vi "Paint Bounding Box.vi"(9 "Camera Image":T3) -> (0 "error out":errorcluster, 1 "Difference":cluster{dbl, dbl}, 2 "Center of Mass":cluster{"X":dbl, "Y":dbl})   [LabVIEW 2016]
uses:
  <vilib>/vision/Image Controls.llb/IMAQ Image.ctl
panel:
  out "Particle Report":T1
  out "Particle Report 2":T1
  out "General Report":T2(array[cluster])
  in  "R/G/B":cluster{"Lower value":i32, "Upper value":i32}[](array[cluster])=[{"Lower value"=0, "Upper value"=40}, {"Lower value"=80, "Upper value"=255}, {"Lower value"=0, "Upper value"=255}]
  out "Particle Report":T2(array[cluster]) {"Orientation" format="%.2f"; "Dimensions"."Height" format="%.2f"; "Dimensions"."Width" format="%.2f"; "Center of Mass"."Y" format="%.2f"; "Center of Mass"."X" format="%.2f"; "Bounding Rect"."Bottom" format="%.2f"; "Bounding Rect"."Right" format="%.2f"; "Bounding Rect"."Top" format="%.2f"; "Bounding Rect"."Left" format="%.2f"; "Number of Holes" format="%.2f"; "Area" format="%.2f"}
  in  "sampleimage":string
  out "Thresholded Image":T3(plugin-control)
  out "Base Image":T3(plugin-control)
  # "difference = width*4"
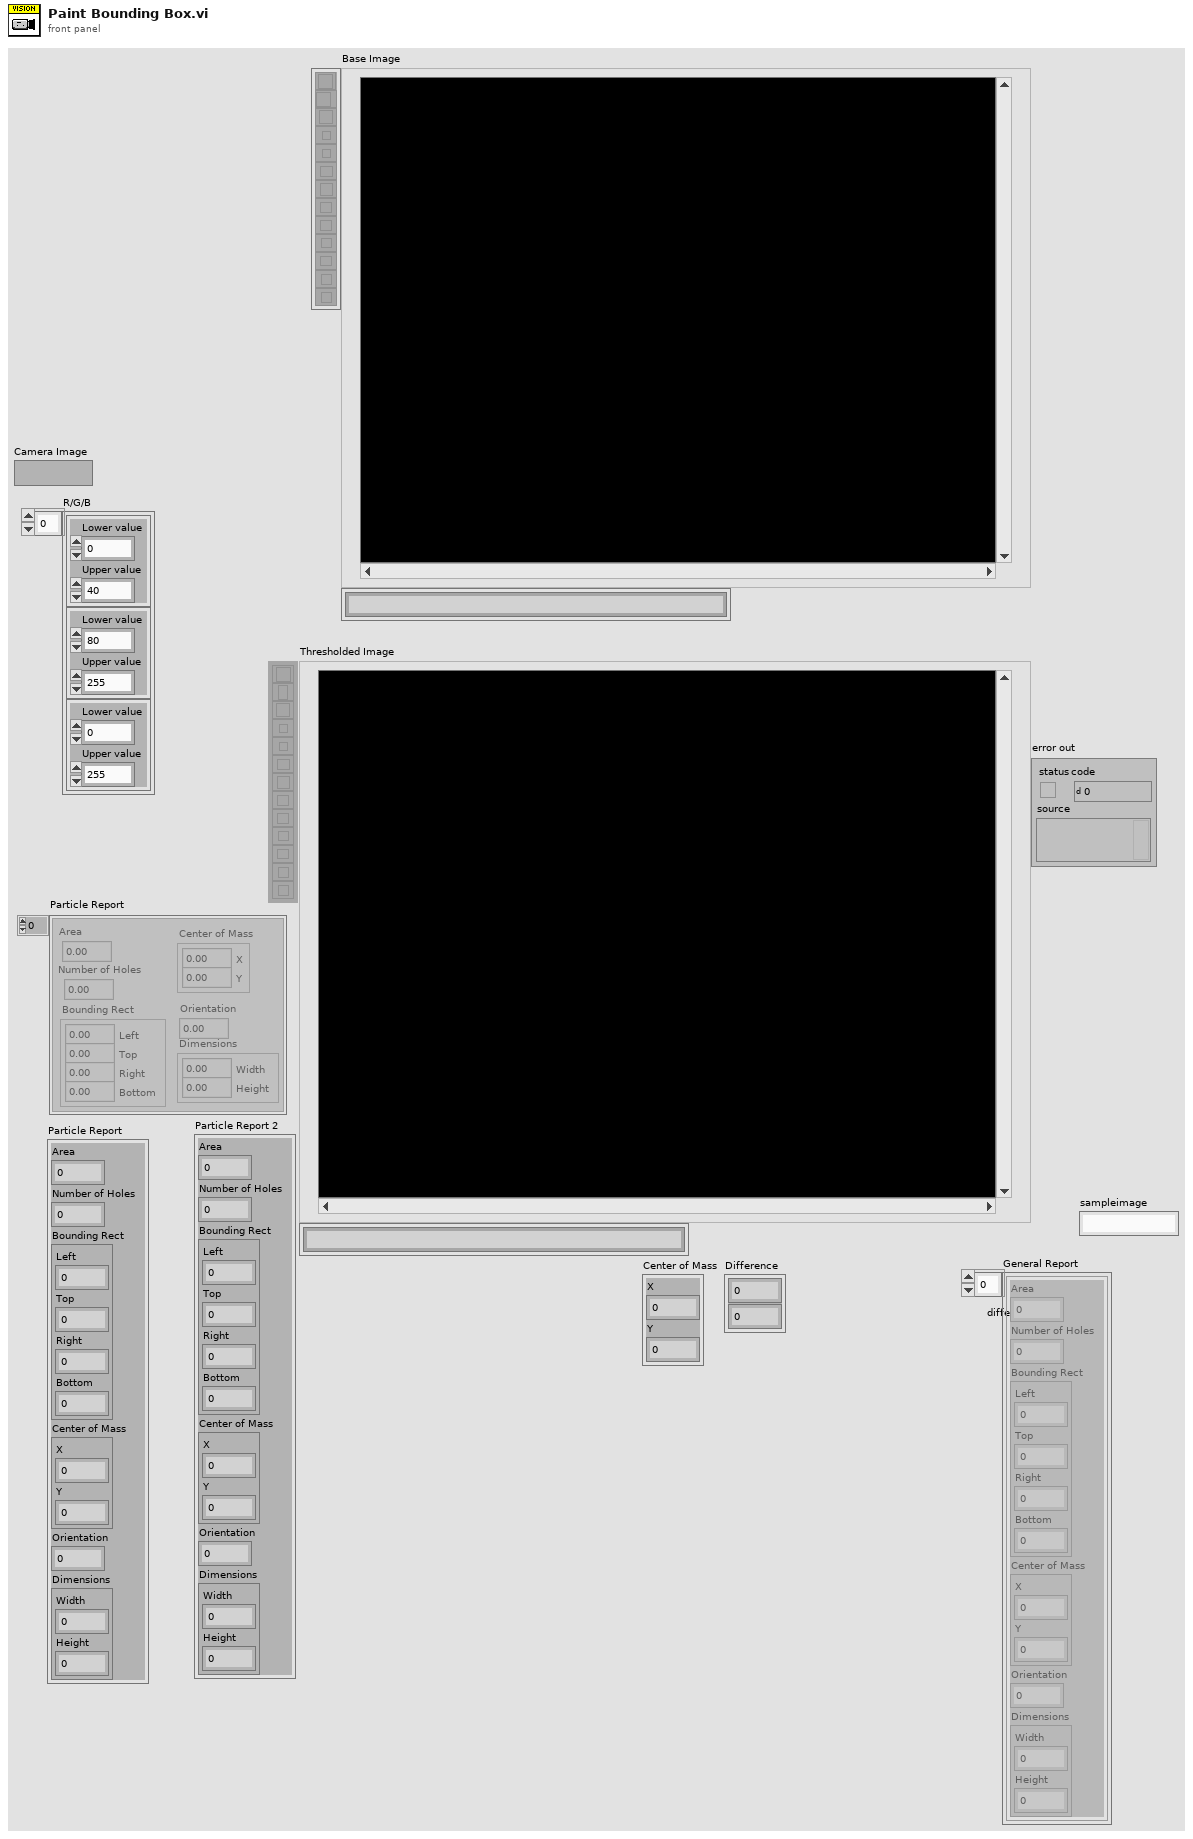
[diagram p1: front panel]
types:
  T1 = cluster{"Area":dbl, "Number of Holes":dbl, "Bounding Rect":cluster{"Left":dbl, "Top":dbl, "Right":dbl, "Bottom":dbl}, "Center of Mass":cluster{"X":dbl, "Y":dbl}, "Orientation":dbl, "Dimensions":cluster{"Width":dbl, "Height":dbl}}
  T2 = cluster{"Area":dbl, "Number of Holes":dbl, "Bounding Rect":cluster{"Left":dbl, "Top":dbl, "Right":dbl, "Bottom":dbl}, "Center of Mass":cluster{"X":dbl, "Y":dbl}, "Orientation":dbl, "Dimensions":cluster{"Width":dbl, "Height":dbl}}[]
  T3 = typedef "IMAQ Image.ctl" = refnum<image>
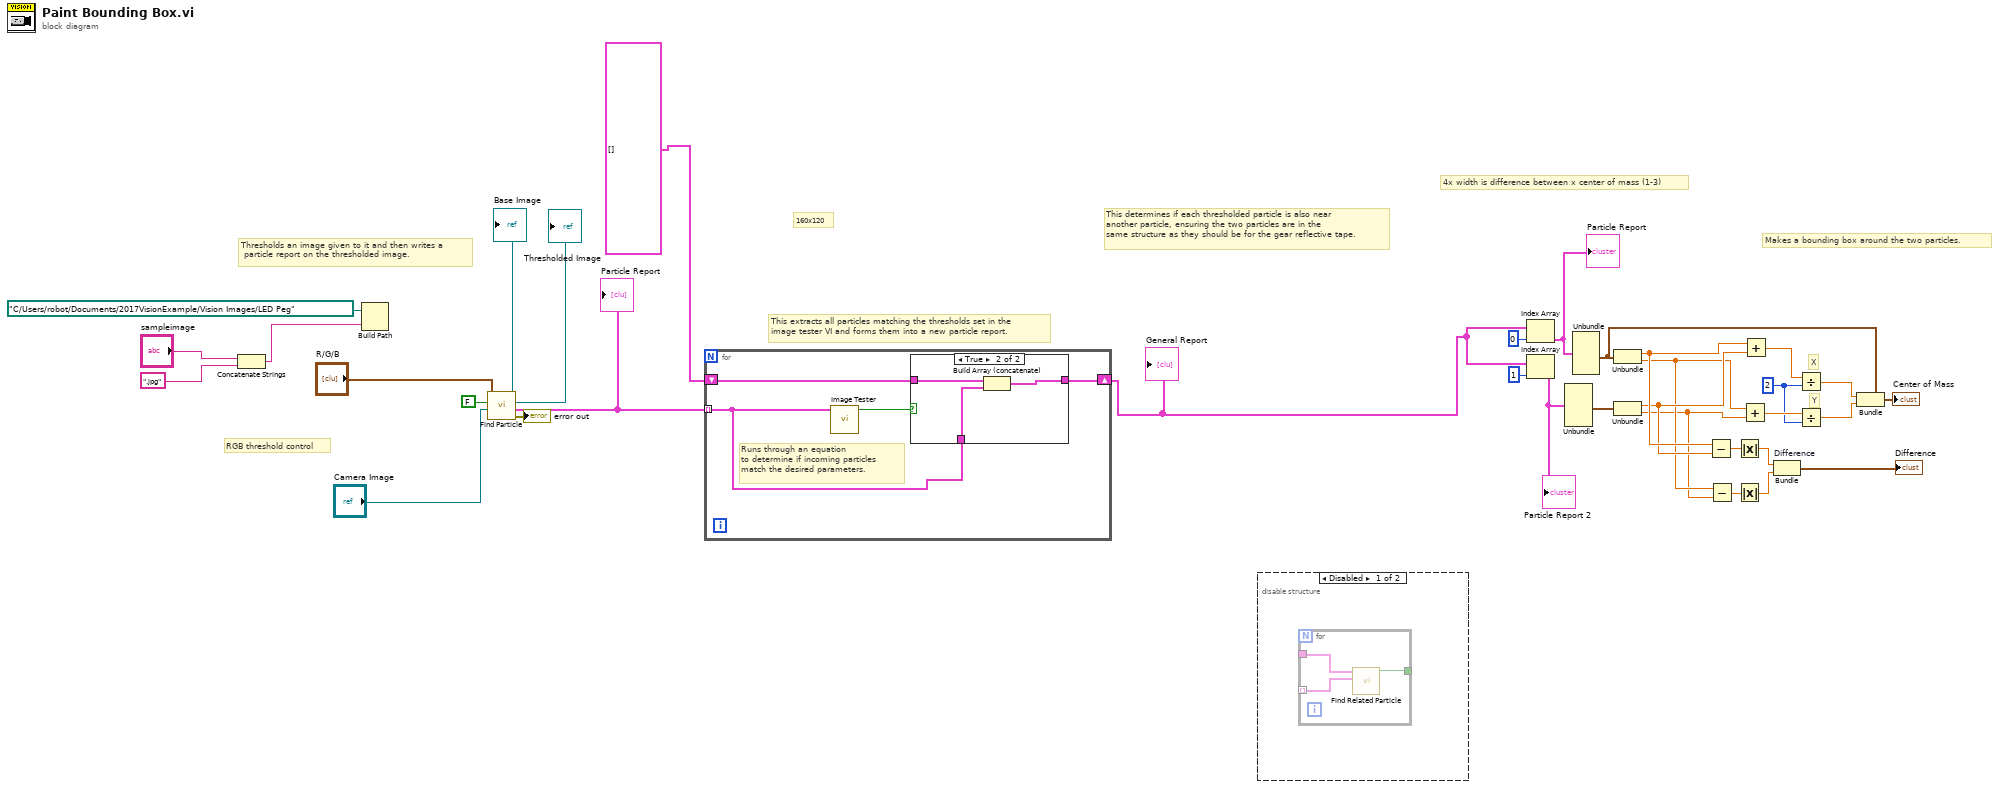
[diagram p0: block diagram]
diagram:
  w15 = 2
  # "Y"
  # "X"
  # "This determines if each thresholded particle is also near \nanother particle, ensuring the two particles are in the \nsame structure as they should be for the gear reflective tape."
  # "Makes a bounding box around the two particles."
  # "4x width is difference between x center of mass (1-3)"
  # "RGB threshold control"
  # "This extracts all particles matching the thresholds set in the \nimage tester VI and forms them into a new particle report."
  # "Thresholds an image given to it and then writes a\n particle report on the thresholded image."
  # "160x120"
  n1 = Concatenate Strings("sampleimage", ".jpg" ("string")) -> (w26:string)
  n2 = Build Path(base path=path "C:/Users/robot/Documents/2017VisionExample/Vision Images/LED Peg", name or relative path=w26) -> ()  [unwired: 1 out]
  n3 = call "Find Particle.vi"("Camera Image"="Camera Image", "From File"=FALSE, "R/G/B"="R/G/B") -> ("error out"=→"error out":errorcluster, "Particle Report"=w32:T2, "Thresholded Image"=→"Thresholded Image":T3, "Base Image"=→"Base Image":T3)  [unwired: 4 in, 1 out]
  "Particle Report" <- w32
  n4 = for {
    tunnel: w32 -> [w35] mode=indexing
    shift-right: [w38] -> w20
    shift-left: T2 [] ("Particle Report") -> [w37]
    # "Runs through an equation\nto determine if incoming particles \nmatch the desired parameters."
    n5 = call "Image Tester.vi"("Particle Report"=w35) -> ("Positive"=w36:bool)  [unwired: 10 in]
    n6 = case shown="True" w36 {
      tunnel: w35 -> [_ w40]
      tunnel: [w39 w42] -> w38
      tunnel: w37 -> [w39 w41]
      frame False {
      }
      frame True {
        n7 = Build Array (concatenate)(w41, w40) -> (w42:T2)
      }
    }
  }
  "General Report" <- w20
  n8 = disable-structure shown="Disabled" {
    frame Disabled {
      n9 = for {
        tunnel: _ -> [w45]
        tunnel: _ -> [w44] mode=indexing
        tunnel: [w43] -> _
        n10 = call "Find Related Particle.vi"("All Reports"=w44, "Base Report"=w45) -> ("Nearby"=w43:bool)  [unwired: 9 in]
      }
    }
    frame Enabled {
    }
  }
  n11 = Index Array(array=w20, index=0) -> (element=w23:T1)
  "Particle Report" <- w23
  n12 = Index Array(array=w20, index=1) -> (element=w22:T1)
  "Particle Report 2" <- w22
  n13 = Unbundle(w22) -> ("Center of Mass"=w18:cluster{"X":dbl, "Y":dbl})  [unwired: 5 out]
  n14 = Unbundle(w23) -> ("Center of Mass"=w14:cluster{"X":dbl, "Y":dbl})  [unwired: 5 out]
  n15 = Unbundle(w14) -> ("X"=w10:dbl, "Y"=w8:dbl)
  n16 = Unbundle(w18) -> ("X"=w9:dbl, "Y"=w7:dbl)
  n17 = Subtract(x=w10, y=w9) -> (x-y=w6:dbl)
  n18 = Subtract(x=w8, y=w7) -> (x-y=w5:dbl)
  n19 = Absolute Value(x=w6) -> (abs(x)=w4:dbl)
  n20 = Absolute Value(x=w5) -> (abs(x)=w3:dbl)
  n21 = Add(x=w8, y=w7) -> (x+y=w16:dbl)
  n22 = Add(x=w10, y=w9) -> (x+y=w17:dbl)
  n23 = Bundle "Difference"(w4, w3) -> (→"Difference":cluster{dbl, dbl})  [unwired: 1 in]
  n24 = Divide(x=w17, y=w15) -> (x/y=w13:dbl)
  n25 = Divide(x=w16, y=w15) -> (x/y=w12:dbl)
  n26 = Bundle(cluster=w14, "X"=w13, "Y"=w12) -> (→"Center of Mass":cluster{"X":dbl, "Y":dbl})
